vi "AddTargetsConfigurationFile.vi"(8 "error in (no error)":errorcluster, 11 "VeriStandTestCase in":refnum<class "VeriStandTestCase.lvclass">) -> (0 "error out":errorcluster, 3 "VeriStandTestCase out":refnum<class "VeriStandTestCase.lvclass">)   [LabVIEW 2016, in "VeriStandTestCase.lvclass"]
uses:
  VeriStandTestCase.lvclass
  VeriStandTestCase.lvclass/VeriStandTestCase.ctl
  <userlib>/_OpenG.lib/file/file.llb/File Exists - Scalar__ogtk.vi
  VeriStandTestUtilities/VeriStandTestUtilities.lvlib
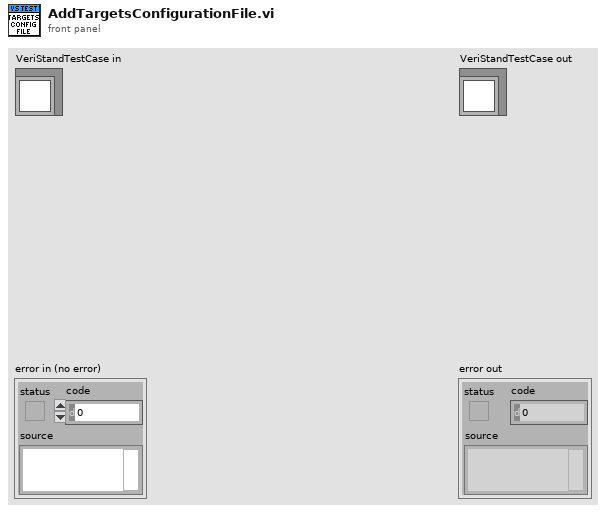
[diagram p1: front panel]
types:
  T1 = typedef "VeriStandTestUtilities.lvlib/TargetsConfiguration.ctl" = cluster{"Supported Targets":cluster{"IP Address / Hostname":string, "Target Platform":T2}[], "Active Configuration":T2}
  T2 = typedef "TargetPlatform.ctl" = enum16{"Windows", "Linux64CRIO", "Linux64PXI", "LinuxARM", "PharLap"}
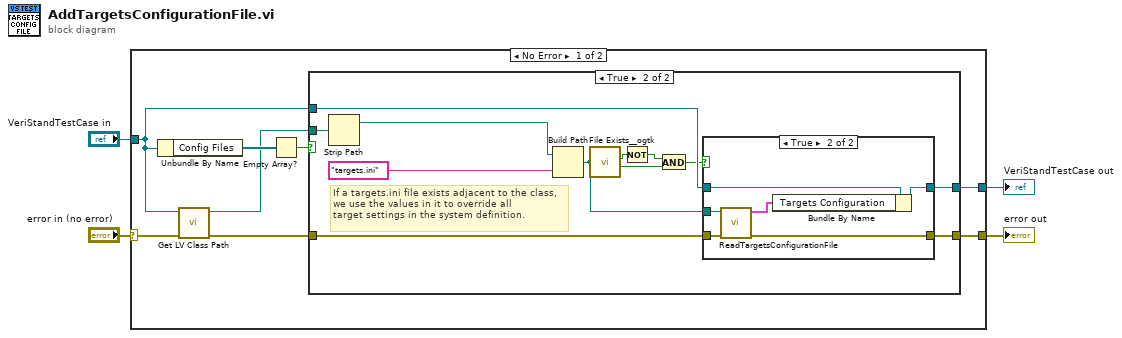
[diagram p0: block diagram]
diagram:
  n1 = case shown="No Error" "error in (no error)" {
    selector: "error in (no error)" -> [w7 w36]
    tunnel: [w11 w36] -> w3
    tunnel: [w12 w35] -> w1
    tunnel: "VeriStandTestCase in" -> [w10 w35]
    frame No Error {
      n2 = Unbundle By Name(w10) -> ("Config Files"=w9:path[])
      n3 = call <vilib>:"Get LV Class Path.vi"("error in (no error)"=w7, "object"=w10) -> ("error out"=w6:errorcluster, "class path"=w5:path)  [unwired: 8 in]
      n4 = Empty Array?(array=w9) -> (empty?=w8:bool)
      n5 = case shown="True" w8 {
        tunnel: w5 -> [_ w21]
        tunnel: w10 -> [w14 w20]
        tunnel: [w14 w18] -> w12
        tunnel: w6 -> [w13 w17]
        tunnel: [w13 w16] -> w11
        frame False {
        }
        frame True {
          # "If a targets.ini file exists adjacent to the class,\nwe use the values in it to override all\ntarget settings in the system definition."
          n6 = Strip Path(path=w21) -> (stripped path=w25:path)  [unwired: 1 out]
          n7 = Build Path(base path=w25, name or relative path="targets.ini") -> (appended path=w15:path)
          n8 = call-poly <userlib>:"File Exists__ogtk.vi"("file path"=w15) -> ("is directory"=w24:bool, "exists"=w22:bool)  [unwired: 6 in]
          n9 = Not(x=w24) -> (.not. x?=w23:bool)
          n10 = And(x=w23, y=w22) -> (x .and. y?=w19:bool)
          n11 = case shown="True" w19 {
            tunnel: w20 -> [w27 w34]
            tunnel: [w27 w33] -> w18
            tunnel: w17 -> [w28 w31]
            tunnel: [w28 w32] -> w16
            tunnel: w15 -> [_ w30]
            frame False {
            }
            frame True {
              n12 = call "ReadTargetsConfigurationFile.vi"("error in (no error)"=w31, "targets.ini file"=w30) -> ("error out"=w32:errorcluster, "Targets Configuration"=w29:T1)  [unwired: 8 in]
              n13 = Bundle By Name(cluster=w34, "Targets Configuration"=w29) -> (w33:refnum<class "VeriStandTestCase.lvclass">)
            }
          }
        }
      }
    }
    frame Error {
    }
  }
  "error out" <- w3
  "VeriStandTestCase out" <- w1
